vi "香农编码.vi"() -> ()   [LabVIEW 2020]
panel:
  out "编码效率：":dbl
  out "信源墒":dbl
  out "平均码长：":dbl
  out "编码":string[](array[string])
  out "Pa(Xj)":dbl[](array[numeric])
  out "ki":i32[](array[numeric])
  in  "P(xi)":dbl[](array[numeric])=[0.25, 0.25, 0.2, 0.15, 0.1, 0.05]
  # "香农编码"
  # "要求P(xi)总\n和为1；"
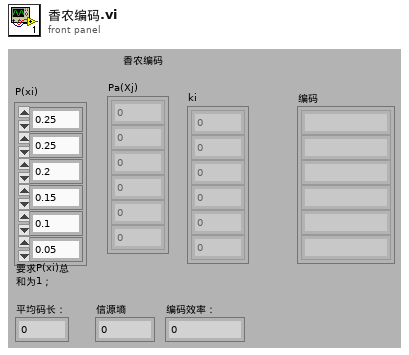
[diagram p1: front panel]
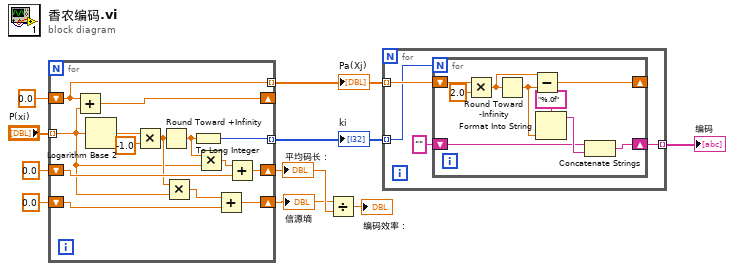
[diagram p0: block diagram]
diagram:
  n1 = for {
    tunnel: "P(xi)" -> [w14] mode=indexing
    tunnel: [w20] -> w7 mode=indexing
    shift-right: [w22] -> _
    shift-left: 0.0 -> [w21]
    tunnel: [w21] -> w8 mode=indexing
    shift-right: [w16] -> w2
    shift-left: 0.0 -> [w19]
    shift-right: [w12] -> w1
    shift-left: 0.0 -> [w11]
    n2 = Add(x=w21, y=w14) -> (x+y=w22:dbl)
    n3 = Logarithm Base 2(1:w14) -> (0:w23:dbl)
    n4 = Multiply(x=w23, y=-1.0) -> (x*y=w15:dbl)
    n5 = Round Toward +Infinity(x=w15) -> (ceil(x): smallest int >= x=w18:dbl)
    n6 = Multiply(x=w15, y=w14) -> (x*y=w13:dbl)
    n7 = To Long Integer(number=w18) -> (32bit integer=w20:i32)
    n8 = Multiply(x=w18, y=w14) -> (x*y=w17:dbl)
    n9 = Add(x=w13, y=w11) -> (x+y=w12:dbl)
    n10 = Add(x=w17, y=w19) -> (x+y=w16:dbl)
  }
  "ki" <- w7
  "Pa(Xj)" <- w8
  "平均码长：" <- w2
  "信源墒" <- w1
  n11 = Divide(x=w1, y=w2) -> (x/y=→"编码效率：":dbl)
  n12 = for {
    tunnel: w8 -> [w28] mode=indexing
    tunnel: w7 -> [w27] mode=indexing
    tunnel: [w26] -> w6 mode=indexing
    n13 = for {
      N: w27 -> [_]
      shift-right: [w35] -> _
      shift-left: w28 -> [w36]
      shift-right: [w30] -> w26
      shift-left: "" -> [w31]
      n14 = Multiply(x=w36, y=2.0) -> (x*y=w34:dbl)
      n15 = Round Toward -Infinity(1:w34) -> (0:w33:dbl)
      n16 = Subtract(x=w34, y=w33) -> (x-y=w35:dbl)
      n17 = Format Into String(format string="%.0f", w33) -> (resulting string=w32:string)  [unwired: 2 in, 1 out]
      n18 = Concatenate Strings(w31, w32) -> (w30:string)
    }
  }
  "编码" <- w6
